vi "Memory.Pointer.Write (unsafe).vi"(8 "error in (no error)":errorcluster, 9 "offset (0)":u64 format="%d bytes", 10 "data":string, 11 "Pointer in":refnum<class "Memory.Pointer.lvclass">) -> (0 "error out":errorcluster, 1 "offset dup":u64 format="%d bytes", 2 "data dup":string, 3 "Pointer out":refnum<class "Memory.Pointer.lvclass">)   [LabVIEW 2016, in "LabVIEW Memory Manager.lvlib" / "Memory.Pointer.lvclass"]
uses:
  Memory.Pointer.lvclass
  Memory.Pointer.lvclass/Memory.Pointer.ctl
  Accessors/Memory.Pointer.Get Address.vi
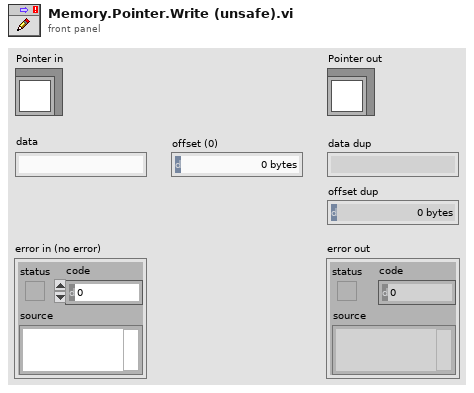
[diagram p1: front panel]
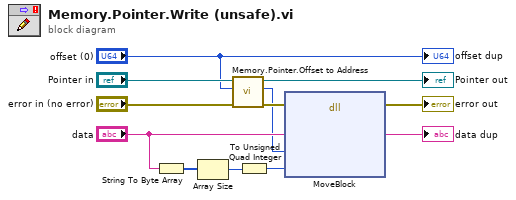
[diagram p0: block diagram]
diagram:
  n1 = String To Byte Array(string="data") -> (unsigned byte array=w12:u8[])
  n2 = Array Size(array=w12) -> (size(s)=w6:i32)
  n3 = call "Memory.Pointer.Offset to Address.vi"("error in (no error)"="error in (no error)", "offset"="offset (0)", "Pointer in"="Pointer in") -> ("error out"=w8:errorcluster, "address"=w7:u64, "Pointer out"=→"Pointer out":refnum<class "Memory.Pointer.lvclass">)  [unwired: 5 in, 1 out]
  n4 = To Unsigned Quad Integer(1:w6) -> (0:w2:u64)
  n5 = dll-call lib="LabVIEW" fn="MoveBlock"(error in=w8, "src pointer"="data", "dst pointer"=w7, "size"=w2) -> (error out=→"error out":errorcluster, "src pointer"=→"data dup":string)  [unwired: 5 in, 1 out]
  "offset dup" <- "offset (0)"
